vi "logger_queue.vi"(8 "error in":errorcluster) -> (0 "error out":errorcluster, 3 "queue out":refnum<queue>)   [LabVIEW 2014]
panel:
  # "Return queue used to log ILEMT data, for use in eg.  stage_calibration.vi, which (if in use) runs concurrently with ilemt_ui.  The format is a 3x11 array of complex double, basically equivalent to the ilemt_ui log file output.  Each row is:\n\n    timestamp entry_type coupling_column_major\n\nThe rows are high rate, low rate, high carriers at low rate.  Unlike in the log file, there is only one high rate entry per low-rate update, the mean of all the individual measurements.  In this case the entry type is simply the row index."
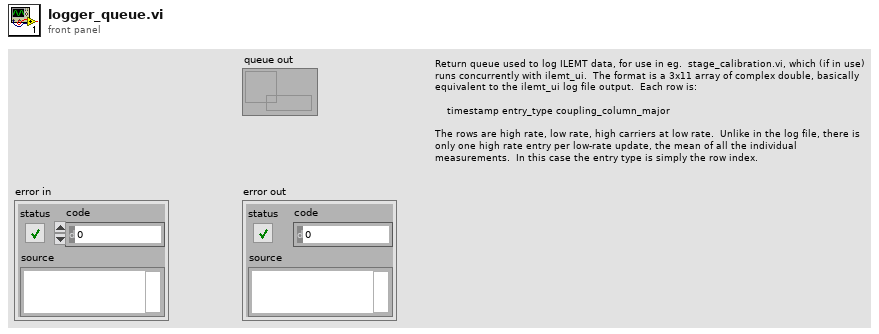
[diagram p1: front panel]
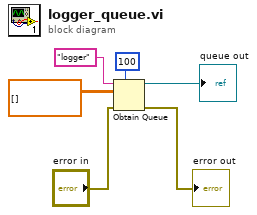
[diagram p0: block diagram]
diagram:
  n1 = Obtain Queue(max queue size (-1, unlimited)=100, name (unnamed)="logger", element data type=cdb[][] [], error in (no error)="error in") -> (queue out=→"queue out":refnum<queue>, error out=→"error out":errorcluster)  [unwired: 1 in, 1 out]
